vi "SeCrTS-DD NS Receiver Pump.vi"(11 "NOT DIS Out":T1) -> ()   [LabVIEW 2022 SP3]
uses:
  Control/SeCrTS-Notifier Ref.ctl
  Globals/SeCrTS-DD globals.vi
  <resource>/objmgr/ni.dex.rc
panel:
  out "x":u32
  out "error out":errorcluster
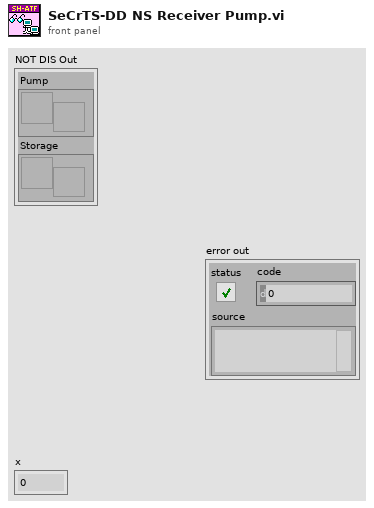
[diagram p1: front panel]
types:
  T1 = typedef "SeCrTS-Notifier Ref.ctl" = cluster{"Pump":refnum<notifier>, "Storage":refnum<notifier>}
  T2 = cluster{"In Progress":bool, "reader url":refnum<k21>, "DI P\nDI S":refnum<queue>[], "Analog Queue":refnum<queue>[], "NOT DIS Out":T1}
  T3 = enum16{"Initialize", "Wait for connection", "Send data", "Exit", "Receive Data"}
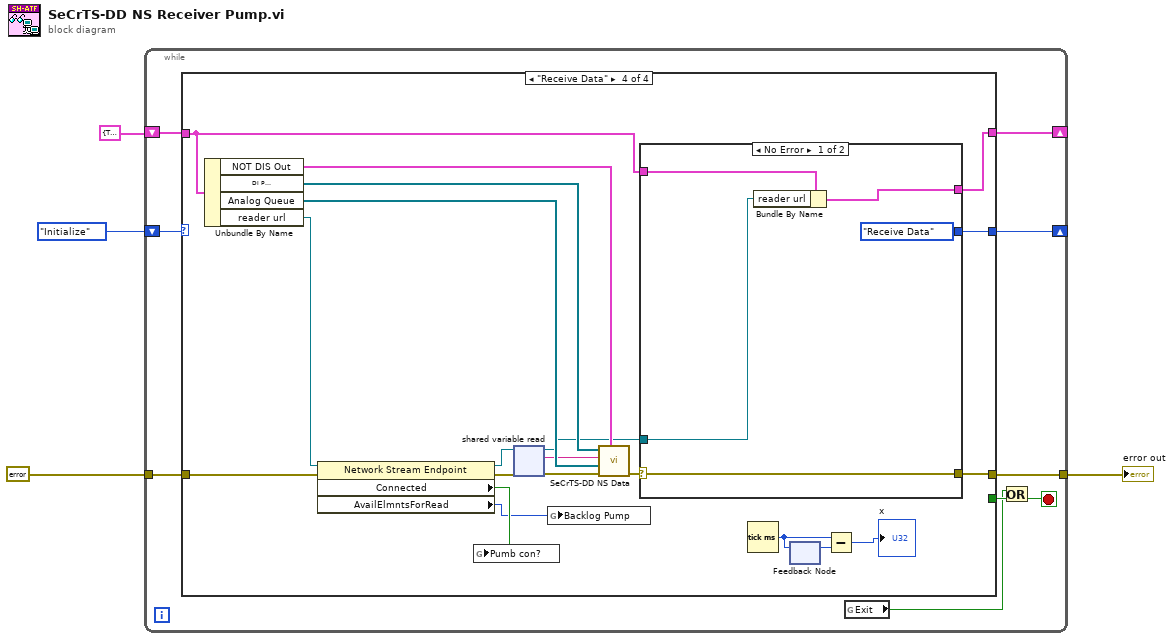
[diagram p0: block diagram]
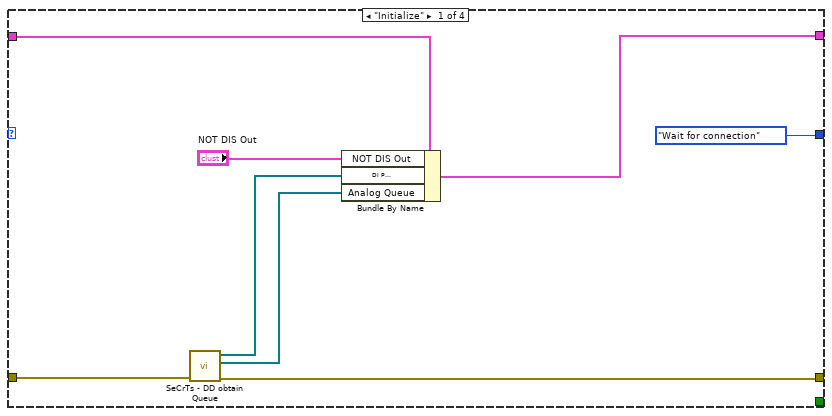
[diagram p2: hidden frame]
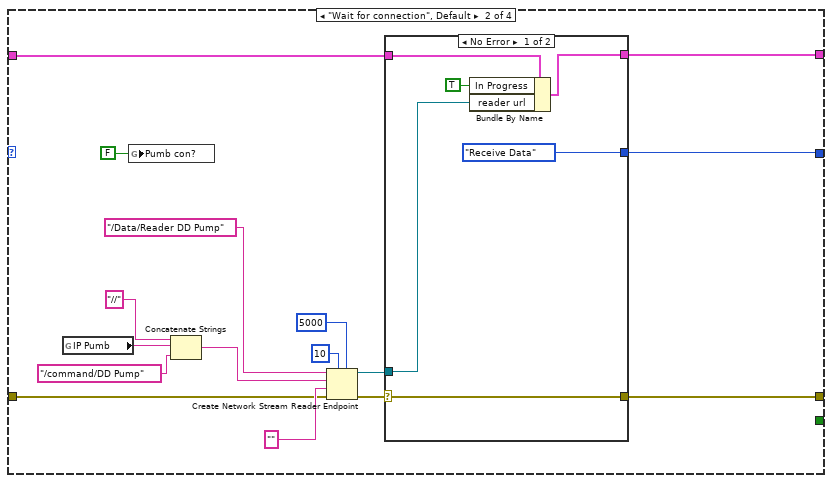
[diagram p3: hidden frame]
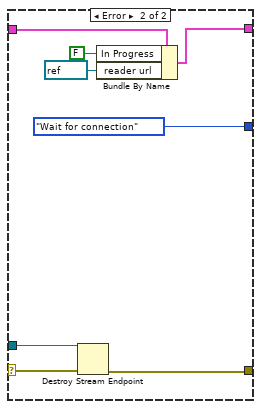
[diagram p4: hidden frame]
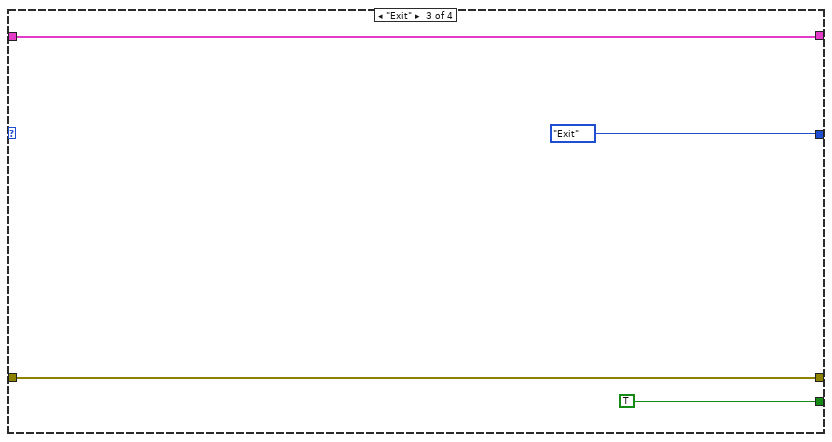
[diagram p5: hidden frame]
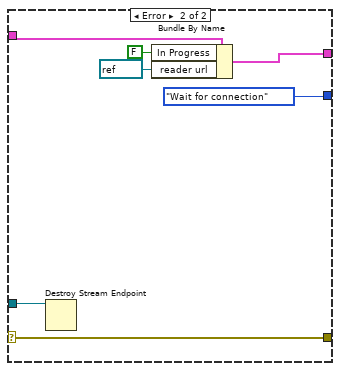
[diagram p6: hidden frame]
diagram:
  n1 = while {
    shift-right: [w11] -> _
    shift-left: T3."Initialize" -> [w13]
    shift-right: [w9] -> _
    shift-left: T2 {"In Progress"=TRUE, "reader url"="", "DI P\nDI S"=[], "Analog Queue"=[], "NOT DIS Out"={"Pump"=refnum, "Storage"=refnum}} -> [w10]
    tunnel: errorcluster {"status"=FALSE, "code"=0, "source"=""} ("error in") -> [w6]
    tunnel: [w5] -> w1
    stop <- w8 stop-if-true
    n2 = case shown="\"Receive Data\"" w13 {
      tunnel: [_ _ TRUE _] -> w12
      tunnel: [T3."Wait for connection" w34 T3."Exit" w61] -> w11
      tunnel: w10 -> [w18 w37 w54 w57]
      tunnel: [w16 w36 w54 w56] -> w9
      tunnel: [w19 w35 w52 w59] -> w5
      tunnel: w6 -> [w20 w24 w52 w68]
      frame "Initialize" {
        n3 = call "SeCrTs - DD obtain Queue.vi"("error in"=w20) -> ("error out"=w19:errorcluster, "AI_V_Data P\nAI_C_Data P\nAO_Data P\nDO_Data P\nACC_Data P\nTC Data P\nDrive_A_C \nDrive_A_D\nAI_C_Data S\nDO_Data S\nAI_V_Rms_P"=w14:refnum<queue>[], "DI P\nDI S"=w15:refnum<queue>[])  [unwired: 8 in]
        n4 = Bundle By Name(cluster=w18, "NOT DIS Out"="NOT DIS Out", "DI P\nDI S"=w15, "Analog Queue"=w14) -> (w16:T2)
      }
      frame "Wait for connection", Default {
        n5 = global read "SeCrTS-DD globals.vi" "IP Pumb"() -> (w27:string)
        n6 = global write "SeCrTS-DD globals.vi" "Pumb con?"(FALSE ("Storage con?")) -> ()
        n7 = Concatenate Strings("//" ("string"), w27, "/command/DD Pump" ("reader url")) -> (w22:string)
        n8 = Create Network Stream Reader Endpoint(5:5000 ("timeout in ms (-1)"), 7:10 ("reader buffer size"), 8:w24, 9:"", 10:w22, 11:"/Data/Reader DD Pump") -> (0:w31:errorcluster, 3:w32:refnum<k21>)  [unwired: 1 in]
        n9 = case shown="No Error" w31 {
          selector: w31 -> [w40 w47]
          tunnel: w37 -> [w43 w51]
          tunnel: w32 -> [w38 w48]
          tunnel: [w41 w50] -> w36
          tunnel: [w40 w46] -> w35
          tunnel: [T3."Receive Data" T3."Wait for connection"] -> w34
          frame No Error {
            n10 = Bundle By Name(cluster=w43, "In Progress"=TRUE, "reader url"=w38) -> (w41:T2)
          }
          frame Error {
            n11 = Destroy Stream Endpoint(8:w47, 11:w48) -> (0:w46:errorcluster)
            n12 = Bundle By Name(cluster=w51, "In Progress"=FALSE, "reader url"=refnum<k21> refnum) -> (w50:T2)
          }
        }
      }
      frame "Exit" {
      }
      frame "Receive Data" {
        n13 = Unbundle By Name(w57) -> ("NOT DIS Out"=w63:T1, "DI P\nDI S"=w66:refnum<queue>[], "Analog Queue"=w65:refnum<queue>[], "reader url"=w58:refnum<k21>)
        n14 = property class="Network Stream Endpoint"(reference=w58, error in=w68) -> (reference out=w75:refnum<k21>, error out=w74:errorcluster, "Connected"=w73:bool, "AvailElmntsForRead"=w69:i32)
        n15 = global write "SeCrTS-DD globals.vi" "Pumb con?"(w73) -> ()
        n16 = shared-variable-read(w75, w74) -> (w60:refnum<k21>, w67:errorcluster, w64:string)  [unwired: 1 in, 1 out]
        n17 = global write "SeCrTS-DD globals.vi" "Backlog Pump"(w69) -> ()
        n18 = call "SeCrTS-DD NS Data.vi"("NOT DIS Out"=w63, "error in"=w67, "AI_V_Data P\nAI_C_Data P\nAO_Data P\nDO_Data P\nACC_Data P\nTC Data P\nDrive_A_C \nDrive_A_D\nAI_C_Data S\nDO_Data S\nAI_V_Rms_P"=w65, "data out"=w64, "DI P\nDI S"=w66) -> ("error out"=w62:errorcluster)  [unwired: 6 in]
        n19 = case shown="No Error" w62 {
          selector: w62 -> [w80 w87]
          tunnel: [w80 w87] -> w59
          tunnel: [T3."Receive Data" T3."Wait for connection"] -> w61
          tunnel: w60 -> [w76 w85]
          tunnel: w57 -> [w77 w84]
          tunnel: [w78 w82] -> w56
          frame No Error {
            n20 = Bundle By Name(cluster=w77, "reader url"=w76) -> (w78:T2)
          }
          frame Error {
            n21 = Destroy Stream Endpoint(11:w85) -> ()  [unwired: 1 in, 1 out]
            n22 = Bundle By Name(cluster=w84, "In Progress"=FALSE, "reader url"=refnum<k21> refnum) -> (w82:T2)
          }
        }
        n23 = Tick Count (ms)() -> (millisecond timer value=w71:u32)
        n24 = feedback #1() -> (w72:u32)  [unwired: 1 in]
        n25 = feedback-in #1(w71) -> ()
        n26 = Subtract(x=w71, y=w72) -> (x-y=→"x":u32)
      }
    }
    n27 = global read "SeCrTS-DD globals.vi" "Exit"() -> (w7:bool)
    n28 = Or(x=w7, y=w12) -> (x .or. y?=w8:bool)
  }
  "error out" <- w1
